vi "Test Free Task.vi"   [LabVIEW 2018]
uses:
  928b0845-a196-4f10-8f33-3f6dc384d574.vi
  <vilib>/addons/_JKI Toolkits/Caraya/classes/Assert/Assert Not Error.vi
  TwinCAT ADS Class/VIs/Data/Read.vi
  <vilib>/addons/_JKI Toolkits/Caraya/classes/Assert/Assert Equal Value and Type_Variant.vi
  <vilib>/addons/_JKI Toolkits/Caraya/classes/Test/Test.lvclass
  <vilib>/addons/_JKI Toolkits/Caraya/classes/Assert/Assert.lvclass
  TwinCAT ADS Class/TwinCAT ADS.lvclass
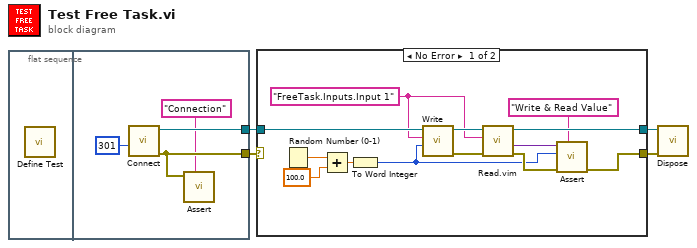
[diagram p0: block diagram]
diagram:
  n1 = flat-sequence {
    tunnel: [w7] -> w3
    tunnel: [w6] -> w4
    frame #0 {
      n2 = call <vilib>:"Define Test.vi"() -> ()  [unwired: 10 in, 2 out]
    }
    frame #1 {
      n3 = call "Connect.vi"("Port"=301) -> ("error out"=w6:errorcluster, "TwinCAT ADS out"=w7:refnum<class "TwinCAT ADS.lvclass">)  [unwired: 9 in]
      n4 = call-poly <vilib>:"Assert.vi"("Label"="Connection", "Not Error?"=w6) -> ()  [unwired: 8 in, 2 out]
    }
  }
  n5 = case shown="No Error" w4 {
    selector: w4 -> [_ w22]
    tunnel: w3 -> [w17 w23]
    tunnel: [w12 w23] -> w2
    tunnel: [w13 w22] -> w1
    frame No Error {
      w10 = "FreeTask.Inputs.Input 1" ("Label")
      n6 = Random Number (0-1)() -> (number: 0 to 1=w16:dbl)
      n7 = Add(x=w16, y=100.0) -> (x+y=w14:dbl)
      n8 = To Word Integer(number=w14) -> (16bit integer=w11:i16)
      n9 = call "Write.vi"("Value"=w11, "Symbol Name"=w10, "TwinCAT ADS in"=w17) -> ("error out"=w18:errorcluster, "TwinCAT ADS out"=w21:refnum<class "TwinCAT ADS.lvclass">)  [unwired: 7 in]
      n10 = call "Read.vim"("error in (no error)"=w18, "Symbol Name"=w10, "TwinCAT ADS in"=w21) -> ("error out"=w20:errorcluster, "Value"=w19:variant, "TwinCAT ADS out"=w12:refnum<class "TwinCAT ADS.lvclass">)  [unwired: 6 in]
      n11 = call-poly <vilib>:"Assert.vi"("Label"="Write & Read Value", "error in (no error)"=w20, "Y"=w11, "X"=w19) -> ("error out"=w13:errorcluster)  [unwired: 6 in, 1 out]
    }
    frame Error {
    }
  }
  n12 = call "Dispose.vi"("error in (no error)"=w1, "TwinCAT ADS in"=w2) -> ()  [unwired: 9 in, 1 out]
